vi "Pos Info.vi"(11 "Echo Info":string) -> (0 "Check Result":bool, 1 "Pos Data":u32, 2 "FC":u8, 3 "Amplifier Num":u8)   [LabVIEW 2014, in "ALPHA5 RS485.lvlib"]
uses:
  ALPHA5 RS485.lvlib
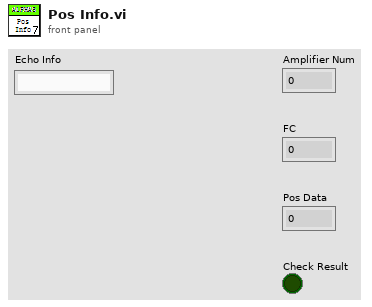
[diagram p1: front panel]
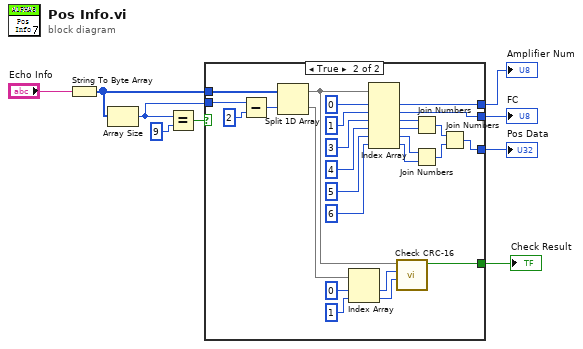
[diagram p0: block diagram]
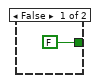
[diagram p2: hidden frame]
diagram:
  n1 = String To Byte Array(string="Echo Info") -> (unsigned byte array=w6:u8[])
  n2 = Array Size(array=w6) -> (size(s)=w5:i32)
  n3 = Equal?(x=w5, y=9) -> (x = y?=w7:bool)
  n4 = case shown="True" w7 {
    tunnel: w6 -> [_ w36]
    tunnel: w5 -> [_ w35]
    tunnel: [FALSE ("Check Result") w27] -> w4
    tunnel: [_ w21] -> w3
    tunnel: [_ w18] -> w2
    tunnel: [_ w11] -> w1
    frame False {
    }
    frame True {
      n5 = Subtract(x=w35, y=2) -> (x-y=w33:i32)
      n6 = Split 1D Array(array=w36, index=w33) -> (first subarray=w22:u8[], second subarray=w32:u8[])
      n7 = Index Array(array=w32, index #1=0 ("index"), index #2=1 ("index")) -> (element #1=w29:u8, element #2=w28:u8)
      n8 = Index Array(array=w22, index #1=0 ("index"), index #2=1 ("index"), index #3=3 ("index"), index #4=4 ("index"), index #5=5 ("index"), index #6=6 ("index")) -> (element #1=w21:u8, element #2=w18:u8, element #3=w17:u8, element #4=w16:u8, element #5=w15:u8, element #6=w14:u8)
      n9 = call "Check CRC-16.vi"("CRC-16-H"=w28, "CRC-16-L"=w29, "Data In"=w22) -> ("Check Result"=w27:bool)  [unwired: 7 in, 1 out]
      n10 = Join Numbers(hi=w17, lo=w16) -> ((hi.lo)=w13:u16)
      n11 = Join Numbers(hi=w15, lo=w14) -> ((hi.lo)=w12:u16)
      n12 = Join Numbers(hi=w13, lo=w12) -> ((hi.lo)=w11:u32)
    }
  }
  "Check Result" <- w4
  "Amplifier Num" <- w3
  "FC" <- w2
  "Pos Data" <- w1
